vi "S4GUI.vi"() -> ()   [LabVIEW 2018] (continued)
            n2694 = call-dynamic "Read AcquisitionA.vi"("error in (no error)"=w6516, "S4ACS_GUI in"=w6518) -> ("error out"=w6521:errorcluster, "Acquisition.lvclass"=w6520:refnum<class "Acquisition.lvclass">, "S4ACS_GUI out"=w6517:refnum<class "S4GUI.lvclass">)  [unwired: 7 in]
            n2695 = call-dynamic "Read Channel.vi"("error in (no error)"=w6521, "Acquisition in"=w6520) -> ("error out"=w6523:errorcluster, "Channel.lvclass"=w6522:refnum<class "Channel.lvclass">, "Acquisition out"=w6529:refnum<class "Acquisition.lvclass">)  [unwired: 7 in]
            n2696 = call-dynamic "Read State Machine.vi"("error in (no error)"=w6523, "Device in"=w6522) -> ("error out"=w6525:errorcluster, "State Machine.lvclass"=w6524:refnum<class "State Machine.lvclass">, "Device out"=w6527:refnum<class "Channel.lvclass">)  [unwired: 7 in]
            n2697 = call "Next State.vi"("error in (no error)"=w6525, "New_State"=u32 80, "State Machine in"=w6524) -> ("error out"=w6528:errorcluster, "State Machine out"=w6526:refnum<class "State Machine.lvclass">)  [unwired: 7 in]
            n2698 = call-dynamic "Write State Machine.vi"("error in (no error)"=w6528, "State Machine.lvclass"=w6526, "Device in"=w6527) -> ("error out"=w6530:errorcluster, "Device out"=w6531:refnum<class "Channel.lvclass">)  [unwired: 7 in]
            n2699 = call-dynamic "Write Channel.vi"("error in (no error)"=w6530, "Channel.lvclass"=w6531, "Acquisition in"=w6529) -> ("error out"=w6513:errorcluster, "Acquisition out"=w6514:refnum<class "Acquisition.lvclass">)  [unwired: 7 in]
            n2700 = call-dynamic "Write Acq_state.vi"("error in (no error)"=w6513, "Acq_state"=u32 0, "Acquisition in"=w6514) -> ("error out"=w6512:errorcluster, "Acquisition out"=w6511:refnum<class "Acquisition.lvclass">)  [unwired: 7 in]
            n2701 = call-dynamic "Write AcquisitionA.vi"("error in (no error)"=w6512, "Acquisition.lvclass"=w6511, "S4ACS_GUI in"=w6517) -> ("error out"=w6499:errorcluster, "S4ACS_GUI out"=w6497:refnum<class "S4GUI.lvclass">)  [unwired: 7 in]
            n2702 = call "Read Instrument.lvclass.vi"("error in (no error)"=w6499, "S4ACS_GUI in"=w6497) -> ("error out"=w6506:errorcluster, "Instrument.lvclass"=w6509:refnum<class "Instrument.lvclass">, "S4ACS_GUI out"=w6510:refnum<class "S4GUI.lvclass">)  [unwired: 7 in]
            n2703 = call "Read WPROT.vi"("error in (no error)"=w6506, "Instrument in"=w6509) -> ("error out"=w6505:errorcluster, "Opt_Selector.lvclass"=w6507:refnum<class "Opt_Selector.lvclass">, "Instrument out"=w6508:refnum<class "Instrument.lvclass">)  [unwired: 7 in]
            n2704 = call-dynamic "Read sequencia_ant.vi"("error in (no error)"=w6505, "Opt_Selector in"=w6507) -> ("error out"=w6501:errorcluster, "sequencia_ant"=w6500:u16, "Opt_Selector out"=w6502:refnum<class "Opt_Selector.lvclass">)  [unwired: 7 in]
            n2705 = call-dynamic "Write sequencia.vi"("error in (no error)"=w6501, "sequencia"=w6500, "Opt_Selector in"=w6502) -> ("error out"=w6490:errorcluster, "Opt_Selector out"=w6491:refnum<class "Opt_Selector.lvclass">)  [unwired: 7 in]
            n2706 = call-dynamic "Read State Machine.vi"("error in (no error)"=w6490, "Device in"=w6491) -> ("error out"=w6493:errorcluster, "State Machine.lvclass"=w6496:refnum<class "State Machine.lvclass">, "Device out"=w6489:refnum<class "Opt_Selector.lvclass">)  [unwired: 7 in]
            n2707 = call "Next State.vi"("error in (no error)"=w6493, "New_State"=10, "State Machine in"=w6496) -> ("error out"=w6492:errorcluster, "State Machine out"=w6495:refnum<class "State Machine.lvclass">)  [unwired: 7 in]
            n2708 = call-dynamic "Write State Machine.vi"("error in (no error)"=w6492, "State Machine.lvclass"=w6495, "Device in"=w6489) -> ("error out"=w6487:errorcluster, "Device out"=w6488:refnum<class "Opt_Selector.lvclass">)  [unwired: 7 in]
            n2709 = call "Write WPROT.vi"("error in (no error)"=w6487, "Opt_Selector.lvclass"=w6488, "Instrument in"=w6508) -> ("error out"=w6504:errorcluster, "Instrument out"=w6503:refnum<class "Instrument.lvclass">)  [unwired: 7 in]
            n2710 = call "Write Instrument.lvclass.vi"("error in (no error)"=w6504, "Instrument.lvclass"=w6503, "S4ACS_GUI in"=w6510) -> ("error out"=w6498:errorcluster, "S4ACS_GUI out"=w6486:refnum<class "S4GUI.lvclass">)  [unwired: 7 in]
          }
          frame Enabled {
            w6535 = FALSE ("Wait Until Done")
            n2711 = call <vilib>:"Application Directory.vi"() -> ("Application Directory"=w6538:path)
            n2712 = Build Path(base path=w6538, name or relative path="MsgAbort1.vi") -> (appended path=w6539:path)
            n2713 = Open VI Reference(vi path=w6539, error in (no error)=w6533) -> (vi reference=w6537:refnum<vi>, error out=w6536:errorcluster)  [unwired: 4 in]
            n2714 = invoke class="VI" method="Run VI"(reference=w6537, error in=w6536, "Wait until done"=w6535, "Auto Dispose Ref"=w6535) -> (error out=w6532:errorcluster)  [unwired: 1 in, 4 out]
          }
        }
      }
      event "Abort ch2": Value Change {
        n2715 = event-data() -> ()  [unwired: 1 in, 6 out]
        n2716 = disable-structure shown="Enabled" {
          disable-tunnel: w6544 -> [w6577 w6592]
          disable-tunnel: w6543 -> [w6575 w6593]
          disable-tunnel: [w6557 w6591] -> w6542
          disable-tunnel: [w6545 w6592] -> w6541
          frame Disabled {
            # "Para movimento \nda lamina retardadora"
            # "Restaura a última sequência de lâminas"
            n2717 = call "Read AcquisitionB.vi"("error in (no error)"=w6575, "S4ACS_GUI in"=w6577) -> ("error out"=w6580:errorcluster, "Acquisition.lvclass"=w6579:refnum<class "Acquisition.lvclass">, "S4ACS_GUI out"=w6576:refnum<class "S4GUI.lvclass">)  [unwired: 7 in]
            n2718 = call-dynamic "Read Channel.vi"("error in (no error)"=w6580, "Acquisition in"=w6579) -> ("error out"=w6582:errorcluster, "Channel.lvclass"=w6581:refnum<class "Channel.lvclass">, "Acquisition out"=w6588:refnum<class "Acquisition.lvclass">)  [unwired: 7 in]
            n2719 = call-dynamic "Read State Machine.vi"("error in (no error)"=w6582, "Device in"=w6581) -> ("error out"=w6584:errorcluster, "State Machine.lvclass"=w6583:refnum<class "State Machine.lvclass">, "Device out"=w6586:refnum<class "Channel.lvclass">)  [unwired: 7 in]
            n2720 = call "Next State.vi"("error in (no error)"=w6584, "New_State"=u32 80, "State Machine in"=w6583) -> ("error out"=w6587:errorcluster, "State Machine out"=w6585:refnum<class "State Machine.lvclass">)  [unwired: 7 in]
            n2721 = call-dynamic "Write State Machine.vi"("error in (no error)"=w6587, "State Machine.lvclass"=w6585, "Device in"=w6586) -> ("error out"=w6589:errorcluster, "Device out"=w6590:refnum<class "Channel.lvclass">)  [unwired: 7 in]
            n2722 = call-dynamic "Write Channel.vi"("error in (no error)"=w6589, "Channel.lvclass"=w6590, "Acquisition in"=w6588) -> ("error out"=w6572:errorcluster, "Acquisition out"=w6573:refnum<class "Acquisition.lvclass">)  [unwired: 7 in]
            n2723 = call-dynamic "Write Acq_state.vi"("error in (no error)"=w6572, "Acq_state"=u32 0, "Acquisition in"=w6573) -> ("error out"=w6571:errorcluster, "Acquisition out"=w6570:refnum<class "Acquisition.lvclass">)  [unwired: 7 in]
            n2724 = call "Write AcquisitionB.vi"("error in (no error)"=w6571, "Acquisition.lvclass"=w6570, "S4ACS_GUI in"=w6576) -> ("error out"=w6558:errorcluster, "S4ACS_GUI out"=w6556:refnum<class "S4GUI.lvclass">)  [unwired: 7 in]
            n2725 = call "Read Instrument.lvclass.vi"("error in (no error)"=w6558, "S4ACS_GUI in"=w6556) -> ("error out"=w6565:errorcluster, "Instrument.lvclass"=w6568:refnum<class "Instrument.lvclass">, "S4ACS_GUI out"=w6569:refnum<class "S4GUI.lvclass">)  [unwired: 7 in]
            n2726 = call "Read WPROT.vi"("error in (no error)"=w6565, "Instrument in"=w6568) -> ("error out"=w6564:errorcluster, "Opt_Selector.lvclass"=w6566:refnum<class "Opt_Selector.lvclass">, "Instrument out"=w6567:refnum<class "Instrument.lvclass">)  [unwired: 7 in]
            n2727 = call-dynamic "Read sequencia_ant.vi"("error in (no error)"=w6564, "Opt_Selector in"=w6566) -> ("error out"=w6560:errorcluster, "sequencia_ant"=w6559:u16, "Opt_Selector out"=w6561:refnum<class "Opt_Selector.lvclass">)  [unwired: 7 in]
            n2728 = call-dynamic "Write sequencia.vi"("error in (no error)"=w6560, "sequencia"=w6559, "Opt_Selector in"=w6561) -> ("error out"=w6549:errorcluster, "Opt_Selector out"=w6550:refnum<class "Opt_Selector.lvclass">)  [unwired: 7 in]
            n2729 = call-dynamic "Read State Machine.vi"("error in (no error)"=w6549, "Device in"=w6550) -> ("error out"=w6552:errorcluster, "State Machine.lvclass"=w6555:refnum<class "State Machine.lvclass">, "Device out"=w6548:refnum<class "Opt_Selector.lvclass">)  [unwired: 7 in]
            n2730 = call "Next State.vi"("error in (no error)"=w6552, "New_State"=10, "State Machine in"=w6555) -> ("error out"=w6551:errorcluster, "State Machine out"=w6554:refnum<class "State Machine.lvclass">)  [unwired: 7 in]
            n2731 = call-dynamic "Write State Machine.vi"("error in (no error)"=w6551, "State Machine.lvclass"=w6554, "Device in"=w6548) -> ("error out"=w6546:errorcluster, "Device out"=w6547:refnum<class "Opt_Selector.lvclass">)  [unwired: 7 in]
            n2732 = call "Write WPROT.vi"("error in (no error)"=w6546, "Opt_Selector.lvclass"=w6547, "Instrument in"=w6567) -> ("error out"=w6563:errorcluster, "Instrument out"=w6562:refnum<class "Instrument.lvclass">)  [unwired: 7 in]
            n2733 = call "Write Instrument.lvclass.vi"("error in (no error)"=w6563, "Instrument.lvclass"=w6562, "S4ACS_GUI in"=w6569) -> ("error out"=w6557:errorcluster, "S4ACS_GUI out"=w6545:refnum<class "S4GUI.lvclass">)  [unwired: 7 in]
          }
          frame Enabled {
            w6595 = FALSE ("Wait Until Done")
            n2734 = call <vilib>:"Application Directory.vi"() -> ("Application Directory"=w6598:path)
            n2735 = Build Path(base path=w6598, name or relative path="MsgAbort2.vi") -> (appended path=w6599:path)
            n2736 = Open VI Reference(vi path=w6599, error in (no error)=w6593) -> (vi reference=w6597:refnum<vi>, error out=w6596:errorcluster)  [unwired: 4 in]
            n2737 = invoke class="VI" method="Run VI"(reference=w6597, error in=w6596, "Wait until done"=w6595, "Auto Dispose Ref"=w6595) -> (error out=w6591:errorcluster)  [unwired: 1 in, 4 out]
          }
        }
      }
      event "Abort ch3": Value Change {
        n2738 = event-data() -> ()  [unwired: 1 in, 6 out]
        n2739 = disable-structure shown="Enabled" {
          disable-tunnel: w6603 -> [w6636 w6651]
          disable-tunnel: w6602 -> [w6634 w6652]
          disable-tunnel: [w6616 w6650] -> w6601
          disable-tunnel: [w6604 w6651] -> w6600
          frame Disabled {
            # "Para movimento \nda lamina retardadora"
            # "Restaura a última sequência de lâminas"
            n2740 = call-dynamic "Read AcquisitionC.vi"("error in (no error)"=w6634, "S4ACS_GUI in"=w6636) -> ("error out"=w6639:errorcluster, "Acquisition.lvclass"=w6638:refnum<class "Acquisition.lvclass">, "S4ACS_GUI out"=w6635:refnum<class "S4GUI.lvclass">)  [unwired: 7 in]
            n2741 = call-dynamic "Read Channel.vi"("error in (no error)"=w6639, "Acquisition in"=w6638) -> ("error out"=w6641:errorcluster, "Channel.lvclass"=w6640:refnum<class "Channel.lvclass">, "Acquisition out"=w6647:refnum<class "Acquisition.lvclass">)  [unwired: 7 in]
            n2742 = call-dynamic "Read State Machine.vi"("error in (no error)"=w6641, "Device in"=w6640) -> ("error out"=w6643:errorcluster, "State Machine.lvclass"=w6642:refnum<class "State Machine.lvclass">, "Device out"=w6645:refnum<class "Channel.lvclass">)  [unwired: 7 in]
            n2743 = call "Next State.vi"("error in (no error)"=w6643, "New_State"=u32 80, "State Machine in"=w6642) -> ("error out"=w6646:errorcluster, "State Machine out"=w6644:refnum<class "State Machine.lvclass">)  [unwired: 7 in]
            n2744 = call-dynamic "Write State Machine.vi"("error in (no error)"=w6646, "State Machine.lvclass"=w6644, "Device in"=w6645) -> ("error out"=w6648:errorcluster, "Device out"=w6649:refnum<class "Channel.lvclass">)  [unwired: 7 in]
            n2745 = call-dynamic "Write Channel.vi"("error in (no error)"=w6648, "Channel.lvclass"=w6649, "Acquisition in"=w6647) -> ("error out"=w6631:errorcluster, "Acquisition out"=w6632:refnum<class "Acquisition.lvclass">)  [unwired: 7 in]
            n2746 = call-dynamic "Write Acq_state.vi"("error in (no error)"=w6631, "Acq_state"=u32 0, "Acquisition in"=w6632) -> ("error out"=w6630:errorcluster, "Acquisition out"=w6629:refnum<class "Acquisition.lvclass">)  [unwired: 7 in]
            n2747 = call-dynamic "Write AcquisitionC.vi"("error in (no error)"=w6630, "Acquisition.lvclass"=w6629, "S4ACS_GUI in"=w6635) -> ("error out"=w6617:errorcluster, "S4ACS_GUI out"=w6615:refnum<class "S4GUI.lvclass">)  [unwired: 7 in]
            n2748 = call "Read Instrument.lvclass.vi"("error in (no error)"=w6617, "S4ACS_GUI in"=w6615) -> ("error out"=w6624:errorcluster, "Instrument.lvclass"=w6627:refnum<class "Instrument.lvclass">, "S4ACS_GUI out"=w6628:refnum<class "S4GUI.lvclass">)  [unwired: 7 in]
            n2749 = call "Read WPROT.vi"("error in (no error)"=w6624, "Instrument in"=w6627) -> ("error out"=w6623:errorcluster, "Opt_Selector.lvclass"=w6625:refnum<class "Opt_Selector.lvclass">, "Instrument out"=w6626:refnum<class "Instrument.lvclass">)  [unwired: 7 in]
            n2750 = call-dynamic "Read sequencia_ant.vi"("error in (no error)"=w6623, "Opt_Selector in"=w6625) -> ("error out"=w6619:errorcluster, "sequencia_ant"=w6618:u16, "Opt_Selector out"=w6620:refnum<class "Opt_Selector.lvclass">)  [unwired: 7 in]
            n2751 = call-dynamic "Write sequencia.vi"("error in (no error)"=w6619, "sequencia"=w6618, "Opt_Selector in"=w6620) -> ("error out"=w6608:errorcluster, "Opt_Selector out"=w6609:refnum<class "Opt_Selector.lvclass">)  [unwired: 7 in]
            n2752 = call-dynamic "Read State Machine.vi"("error in (no error)"=w6608, "Device in"=w6609) -> ("error out"=w6611:errorcluster, "State Machine.lvclass"=w6614:refnum<class "State Machine.lvclass">, "Device out"=w6607:refnum<class "Opt_Selector.lvclass">)  [unwired: 7 in]
            n2753 = call "Next State.vi"("error in (no error)"=w6611, "New_State"=10, "State Machine in"=w6614) -> ("error out"=w6610:errorcluster, "State Machine out"=w6613:refnum<class "State Machine.lvclass">)  [unwired: 7 in]
            n2754 = call-dynamic "Write State Machine.vi"("error in (no error)"=w6610, "State Machine.lvclass"=w6613, "Device in"=w6607) -> ("error out"=w6605:errorcluster, "Device out"=w6606:refnum<class "Opt_Selector.lvclass">)  [unwired: 7 in]
            n2755 = call "Write WPROT.vi"("error in (no error)"=w6605, "Opt_Selector.lvclass"=w6606, "Instrument in"=w6626) -> ("error out"=w6622:errorcluster, "Instrument out"=w6621:refnum<class "Instrument.lvclass">)  [unwired: 7 in]
            n2756 = call "Write Instrument.lvclass.vi"("error in (no error)"=w6622, "Instrument.lvclass"=w6621, "S4ACS_GUI in"=w6628) -> ("error out"=w6616:errorcluster, "S4ACS_GUI out"=w6604:refnum<class "S4GUI.lvclass">)  [unwired: 7 in]
          }
          frame Enabled {
            w6654 = FALSE ("Wait Until Done")
            n2757 = call <vilib>:"Application Directory.vi"() -> ("Application Directory"=w6657:path)
            n2758 = Build Path(base path=w6657, name or relative path="MsgAbort3.vi") -> (appended path=w6658:path)
            n2759 = Open VI Reference(vi path=w6658, error in (no error)=w6652) -> (vi reference=w6656:refnum<vi>, error out=w6655:errorcluster)  [unwired: 4 in]
            n2760 = invoke class="VI" method="Run VI"(reference=w6656, error in=w6655, "Wait until done"=w6654, "Auto Dispose Ref"=w6654) -> (error out=w6650:errorcluster)  [unwired: 1 in, 4 out]
          }
        }
      }
      event "Abort ch4": Value Change {
        n2761 = event-data() -> ()  [unwired: 1 in, 6 out]
        n2762 = disable-structure shown="Enabled" {
          disable-tunnel: w6662 -> [w6695 w6710]
          disable-tunnel: w6661 -> [w6693 w6711]
          disable-tunnel: [w6675 w6709] -> w6660
          disable-tunnel: [w6663 w6710] -> w6659
          frame Disabled {
            # "Para movimento \nda lamina retardadora"
            # "Restaura a última sequência de lâminas"
            n2763 = call-dynamic "Read AcquisitionD.vi"("error in (no error)"=w6693, "S4ACS_GUI in"=w6695) -> ("error out"=w6698:errorcluster, "Acquisition.lvclass"=w6697:refnum<class "Acquisition.lvclass">, "S4ACS_GUI out"=w6694:refnum<class "S4GUI.lvclass">)  [unwired: 7 in]
            n2764 = call-dynamic "Read Channel.vi"("error in (no error)"=w6698, "Acquisition in"=w6697) -> ("error out"=w6700:errorcluster, "Channel.lvclass"=w6699:refnum<class "Channel.lvclass">, "Acquisition out"=w6706:refnum<class "Acquisition.lvclass">)  [unwired: 7 in]
            n2765 = call-dynamic "Read State Machine.vi"("error in (no error)"=w6700, "Device in"=w6699) -> ("error out"=w6702:errorcluster, "State Machine.lvclass"=w6701:refnum<class "State Machine.lvclass">, "Device out"=w6704:refnum<class "Channel.lvclass">)  [unwired: 7 in]
            n2766 = call "Next State.vi"("error in (no error)"=w6702, "New_State"=u32 80, "State Machine in"=w6701) -> ("error out"=w6705:errorcluster, "State Machine out"=w6703:refnum<class "State Machine.lvclass">)  [unwired: 7 in]
            n2767 = call-dynamic "Write State Machine.vi"("error in (no error)"=w6705, "State Machine.lvclass"=w6703, "Device in"=w6704) -> ("error out"=w6707:errorcluster, "Device out"=w6708:refnum<class "Channel.lvclass">)  [unwired: 7 in]
            n2768 = call-dynamic "Write Channel.vi"("error in (no error)"=w6707, "Channel.lvclass"=w6708, "Acquisition in"=w6706) -> ("error out"=w6690:errorcluster, "Acquisition out"=w6691:refnum<class "Acquisition.lvclass">)  [unwired: 7 in]
            n2769 = call-dynamic "Write Acq_state.vi"("error in (no error)"=w6690, "Acq_state"=u32 0, "Acquisition in"=w6691) -> ("error out"=w6689:errorcluster, "Acquisition out"=w6688:refnum<class "Acquisition.lvclass">)  [unwired: 7 in]
            n2770 = call-dynamic "Write AcquisitionD.vi"("error in (no error)"=w6689, "Acquisition.lvclass"=w6688, "S4ACS_GUI in"=w6694) -> ("error out"=w6676:errorcluster, "S4ACS_GUI out"=w6674:refnum<class "S4GUI.lvclass">)  [unwired: 7 in]
            n2771 = call "Read Instrument.lvclass.vi"("error in (no error)"=w6676, "S4ACS_GUI in"=w6674) -> ("error out"=w6683:errorcluster, "Instrument.lvclass"=w6686:refnum<class "Instrument.lvclass">, "S4ACS_GUI out"=w6687:refnum<class "S4GUI.lvclass">)  [unwired: 7 in]
            n2772 = call "Read WPROT.vi"("error in (no error)"=w6683, "Instrument in"=w6686) -> ("error out"=w6682:errorcluster, "Opt_Selector.lvclass"=w6684:refnum<class "Opt_Selector.lvclass">, "Instrument out"=w6685:refnum<class "Instrument.lvclass">)  [unwired: 7 in]
            n2773 = call-dynamic "Read sequencia_ant.vi"("error in (no error)"=w6682, "Opt_Selector in"=w6684) -> ("error out"=w6678:errorcluster, "sequencia_ant"=w6677:u16, "Opt_Selector out"=w6679:refnum<class "Opt_Selector.lvclass">)  [unwired: 7 in]
            n2774 = call-dynamic "Write sequencia.vi"("error in (no error)"=w6678, "sequencia"=w6677, "Opt_Selector in"=w6679) -> ("error out"=w6667:errorcluster, "Opt_Selector out"=w6668:refnum<class "Opt_Selector.lvclass">)  [unwired: 7 in]
            n2775 = call-dynamic "Read State Machine.vi"("error in (no error)"=w6667, "Device in"=w6668) -> ("error out"=w6670:errorcluster, "State Machine.lvclass"=w6673:refnum<class "State Machine.lvclass">, "Device out"=w6666:refnum<class "Opt_Selector.lvclass">)  [unwired: 7 in]
            n2776 = call "Next State.vi"("error in (no error)"=w6670, "New_State"=10, "State Machine in"=w6673) -> ("error out"=w6669:errorcluster, "State Machine out"=w6672:refnum<class "State Machine.lvclass">)  [unwired: 7 in]
            n2777 = call-dynamic "Write State Machine.vi"("error in (no error)"=w6669, "State Machine.lvclass"=w6672, "Device in"=w6666) -> ("error out"=w6664:errorcluster, "Device out"=w6665:refnum<class "Opt_Selector.lvclass">)  [unwired: 7 in]
            n2778 = call "Write WPROT.vi"("error in (no error)"=w6664, "Opt_Selector.lvclass"=w6665, "Instrument in"=w6685) -> ("error out"=w6681:errorcluster, "Instrument out"=w6680:refnum<class "Instrument.lvclass">)  [unwired: 7 in]
            n2779 = call "Write Instrument.lvclass.vi"("error in (no error)"=w6681, "Instrument.lvclass"=w6680, "S4ACS_GUI in"=w6687) -> ("error out"=w6675:errorcluster, "S4ACS_GUI out"=w6663:refnum<class "S4GUI.lvclass">)  [unwired: 7 in]
          }
          frame Enabled {
            w6713 = FALSE ("Wait Until Done")
            n2780 = call <vilib>:"Application Directory.vi"() -> ("Application Directory"=w6716:path)
            n2781 = Build Path(base path=w6716, name or relative path="MsgAbort4.vi") -> (appended path=w6717:path)
            n2782 = Open VI Reference(vi path=w6717, error in (no error)=w6711) -> (vi reference=w6715:refnum<vi>, error out=w6714:errorcluster)  [unwired: 4 in]
            n2783 = invoke class="VI" method="Run VI"(reference=w6715, error in=w6714, "Wait until done"=w6713, "Auto Dispose Ref"=w6713) -> (error out=w6709:errorcluster)  [unwired: 1 in, 4 out]
          }
        }
      }
      event "Exposure Time": Value Change {
        n2784 = event-data() -> ()  [unwired: 1 in, 4 out]
        n2785 = call-dynamic "Read AcquisitionA.vi"("error in (no error)"=w6736, "S4ACS_GUI in"=w6737) -> ("error out"=w6734:errorcluster, "Acquisition.lvclass"=w6735:refnum<class "Acquisition.lvclass">, "S4ACS_GUI out"=w6731:refnum<class "S4GUI.lvclass">)  [unwired: 7 in]
        n2786 = call-dynamic "Read Channel.vi"("error in (no error)"=w6734, "Acquisition in"=w6735) -> ("error out"=w6720:errorcluster, "Channel.lvclass"=w6721:refnum<class "Channel.lvclass">, "Acquisition out"=w6733:refnum<class "Acquisition.lvclass">)  [unwired: 7 in]
        n2787 = call-dynamic "Read Interface.vi"("error in (no error)"=w6720, "Channel in"=w6721) -> ("error out"=w6727:errorcluster, "Interface.lvclass"=w6728:refnum<class "Interface.lvclass">, "Channel out"=w6725:refnum<class "Channel.lvclass">)  [unwired: 7 in]
        n2788 = call "Write Exposure Time.vi"("error in (no error)"=w6727, "Exposure Time"="Exposure Time", "Interface in"=w6728) -> ("error out"=w6722:errorcluster, "Interface out"=w6726:refnum<class "Interface.lvclass">)  [unwired: 7 in]
        n2789 = call-dynamic "Write Interface.vi"("error in (no error)"=w6722, "Interface.lvclass"=w6726, "Channel in"=w6725) -> ("error out"=w6723:errorcluster, "Channel out"=w6724:refnum<class "Channel.lvclass">)  [unwired: 7 in]
        n2790 = call-dynamic "Write Channel.vi"("error in (no error)"=w6723, "Channel.lvclass"=w6724, "Acquisition in"=w6733) -> ("error out"=w6730:errorcluster, "Acquisition out"=w6732:refnum<class "Acquisition.lvclass">)  [unwired: 7 in]
        n2791 = call-dynamic "Write AcquisitionA.vi"("error in (no error)"=w6730, "Acquisition.lvclass"=w6732, "S4ACS_GUI in"=w6731) -> ("error out"=w6729:errorcluster, "S4ACS_GUI out"=w6718:refnum<class "S4GUI.lvclass">)  [unwired: 7 in]
      }
      event "SyncBox": Value Change {
        n2792 = event-data() -> ()  [unwired: 1 in, 4 out]
        n2793 = call-dynamic "Read Sync Box.lvclass.vi"("error in (no error)"=w6740, "SPARC4_AC in"=w6741) -> ("error out"=w6756:errorcluster, "Sync Box.lvclass"=w6757:refnum<class "Sync Box.lvclass">, "SPARC4_AC out"=w6745:refnum<class "S4GUI.lvclass">)  [unwired: 7 in]
        n2794 = call-dynamic "Read Trigger.lvclass.vi"("error in (no error)"=w6756, "Sync Box in"=w6757) -> ("error out"=w6754:errorcluster, "Trigger.lvclass"=w6755:refnum<class "Trigger.lvclass">, "Sync Box out"=w6748:refnum<class "Sync Box.lvclass">)  [unwired: 7 in]
        n2795 = call-dynamic "Read State Machine.vi"("error in (no error)"=w6754, "Device in"=w6755) -> ("error out"=w6752:errorcluster, "State Machine.lvclass"=w6753:refnum<class "State Machine.lvclass">, "Device out"=w6749:refnum<class "Trigger.lvclass">)  [unwired: 7 in]
        n2796 = call "Next State.vi"("error in (no error)"=w6752, "New_State"=u32 1, "State Machine in"=w6753) -> ("error out"=w6747:errorcluster, "State Machine out"=w6750:refnum<class "State Machine.lvclass">)  [unwired: 7 in]
        n2797 = call-dynamic "Write State Machine.vi"("error in (no error)"=w6747, "State Machine.lvclass"=w6750, "Device in"=w6749) -> ("error out"=w6743:errorcluster, "Device out"=w6742:refnum<class "Trigger.lvclass">)  [unwired: 7 in]
        n2798 = call-dynamic "Write Trigger.lvclass.vi"("error in (no error)"=w6743, "Trigger.lvclass"=w6742, "Sync Box in"=w6748) -> ("error out"=w6744:errorcluster, "Sync Box out"=w6746:refnum<class "Sync Box.lvclass">)  [unwired: 7 in]
        n2799 = call-dynamic "Write Sync Box.lvclass.vi"("error in (no error)"=w6744, "Sync Box.lvclass"=w6746, "SPARC4_AC in"=w6745) -> ("error out"=w6739:errorcluster, "SPARC4_AC out"=w6738:refnum<class "S4GUI.lvclass">)  [unwired: 7 in]
      }
      event "Fire manual", "Fire": Value Change {
        n2800 = event-data() -> ()  [unwired: 1 in, 4 out]
        n2801 = call-dynamic "Read Sync Box.lvclass.vi"("error in (no error)"=w6760, "SPARC4_AC in"=w6761) -> ("error out"=w6776:errorcluster, "Sync Box.lvclass"=w6777:refnum<class "Sync Box.lvclass">, "SPARC4_AC out"=w6765:refnum<class "S4GUI.lvclass">)  [unwired: 7 in]
        n2802 = call-dynamic "Read Trigger.lvclass.vi"("error in (no error)"=w6776, "Sync Box in"=w6777) -> ("error out"=w6774:errorcluster, "Trigger.lvclass"=w6775:refnum<class "Trigger.lvclass">, "Sync Box out"=w6768:refnum<class "Sync Box.lvclass">)  [unwired: 7 in]
        n2803 = call-dynamic "Read State Machine.vi"("error in (no error)"=w6774, "Device in"=w6775) -> ("error out"=w6772:errorcluster, "State Machine.lvclass"=w6773:refnum<class "State Machine.lvclass">, "Device out"=w6769:refnum<class "Trigger.lvclass">)  [unwired: 7 in]
        n2804 = call "Next State.vi"("error in (no error)"=w6772, "New_State"=u32 40, "State Machine in"=w6773) -> ("error out"=w6767:errorcluster, "State Machine out"=w6770:refnum<class "State Machine.lvclass">)  [unwired: 7 in]
        n2805 = call-dynamic "Write State Machine.vi"("error in (no error)"=w6767, "State Machine.lvclass"=w6770, "Device in"=w6769) -> ("error out"=w6763:errorcluster, "Device out"=w6762:refnum<class "Trigger.lvclass">)  [unwired: 7 in]
        n2806 = call-dynamic "Write Trigger.lvclass.vi"("error in (no error)"=w6763, "Trigger.lvclass"=w6762, "Sync Box in"=w6768) -> ("error out"=w6764:errorcluster, "Sync Box out"=w6766:refnum<class "Sync Box.lvclass">)  [unwired: 7 in]
        n2807 = call-dynamic "Write Sync Box.lvclass.vi"("error in (no error)"=w6764, "Sync Box.lvclass"=w6766, "SPARC4_AC in"=w6765) -> ("error out"=w6759:errorcluster, "SPARC4_AC out"=w6758:refnum<class "S4GUI.lvclass">)  [unwired: 7 in]
      }
      event "Select Trigger Mode": Value Change {
        n2808 = event-data() -> ("NewVal"=w6779:bool)  [unwired: 1 in, 2 out]
        n2809 = call-dynamic "Read Sync Box.lvclass.vi"("error in (no error)"=w6787, "SPARC4_AC in"=w6788) -> ("error out"=w6799:errorcluster, "Sync Box.lvclass"=w6800:refnum<class "Sync Box.lvclass">, "SPARC4_AC out"=w6792:refnum<class "S4GUI.lvclass">)  [unwired: 7 in]
        n2810 = call-dynamic "Read Trigger.lvclass.vi"("error in (no error)"=w6799, "Sync Box in"=w6800) -> ("error out"=w6780:errorcluster, "Trigger.lvclass"=w6783:refnum<class "Trigger.lvclass">, "Sync Box out"=w6795:refnum<class "Sync Box.lvclass">)  [unwired: 7 in]
        n2811 = call-dynamic "Write Trigger Mode Target.vi"("error in (no error)"=w6780, "Trigger Mode Target"=w6779, "Trigger in"=w6783) -> ("error out"=w6781:errorcluster, "Trigger out"=w6782:refnum<class "Trigger.lvclass">)  [unwired: 7 in]
        n2812 = call-dynamic "Read State Machine.vi"("error in (no error)"=w6781, "Device in"=w6782) -> ("error out"=w6784:errorcluster, "State Machine.lvclass"=w6785:refnum<class "State Machine.lvclass">, "Device out"=w6796:refnum<class "Trigger.lvclass">)  [unwired: 7 in]
        n2813 = call "Next State.vi"("error in (no error)"=w6784, "New_State"=u32 30, "State Machine in"=w6785) -> ("error out"=w6794:errorcluster, "State Machine out"=w6797:refnum<class "State Machine.lvclass">)  [unwired: 7 in]
        n2814 = call-dynamic "Write State Machine.vi"("error in (no error)"=w6794, "State Machine.lvclass"=w6797, "Device in"=w6796) -> ("error out"=w6790:errorcluster, "Device out"=w6789:refnum<class "Trigger.lvclass">)  [unwired: 7 in]
        n2815 = call-dynamic "Write Trigger.lvclass.vi"("error in (no error)"=w6790, "Trigger.lvclass"=w6789, "Sync Box in"=w6795) -> ("error out"=w6791:errorcluster, "Sync Box out"=w6793:refnum<class "Sync Box.lvclass">)  [unwired: 7 in]
        n2816 = call-dynamic "Write Sync Box.lvclass.vi"("error in (no error)"=w6791, "Sync Box.lvclass"=w6793, "SPARC4_AC in"=w6792) -> ("error out"=w6786:errorcluster, "SPARC4_AC out"=w6778:refnum<class "S4GUI.lvclass">)  [unwired: 7 in]
      }
      event "Set SyncBox": Value Change {
        n2817 = event-data() -> ()  [unwired: 1 in, 4 out]
        n2818 = call-dynamic "Read Sync Box.lvclass.vi"("error in (no error)"=w6803, "SPARC4_AC in"=w6804) -> ("error out"=w6819:errorcluster, "Sync Box.lvclass"=w6820:refnum<class "Sync Box.lvclass">, "SPARC4_AC out"=w6808:refnum<class "S4GUI.lvclass">)  [unwired: 7 in]
        n2819 = call-dynamic "Read Trigger.lvclass.vi"("error in (no error)"=w6819, "Sync Box in"=w6820) -> ("error out"=w6817:errorcluster, "Trigger.lvclass"=w6818:refnum<class "Trigger.lvclass">, "Sync Box out"=w6811:refnum<class "Sync Box.lvclass">)  [unwired: 7 in]
        n2820 = call-dynamic "Read State Machine.vi"("error in (no error)"=w6817, "Device in"=w6818) -> ("error out"=w6815:errorcluster, "State Machine.lvclass"=w6816:refnum<class "State Machine.lvclass">, "Device out"=w6812:refnum<class "Trigger.lvclass">)  [unwired: 7 in]
        n2821 = call "Next State.vi"("error in (no error)"=w6815, "New_State"=u32 10, "State Machine in"=w6816) -> ("error out"=w6810:errorcluster, "State Machine out"=w6813:refnum<class "State Machine.lvclass">)  [unwired: 7 in]
        n2822 = call-dynamic "Write State Machine.vi"("error in (no error)"=w6810, "State Machine.lvclass"=w6813, "Device in"=w6812) -> ("error out"=w6806:errorcluster, "Device out"=w6805:refnum<class "Trigger.lvclass">)  [unwired: 7 in]
        n2823 = call-dynamic "Write Trigger.lvclass.vi"("error in (no error)"=w6806, "Trigger.lvclass"=w6805, "Sync Box in"=w6811) -> ("error out"=w6807:errorcluster, "Sync Box out"=w6809:refnum<class "Sync Box.lvclass">)  [unwired: 7 in]
        n2824 = call-dynamic "Write Sync Box.lvclass.vi"("error in (no error)"=w6807, "Sync Box.lvclass"=w6809, "SPARC4_AC in"=w6808) -> ("error out"=w6802:errorcluster, "SPARC4_AC out"=w6801:refnum<class "S4GUI.lvclass">)  [unwired: 7 in]
      }
      event "Cooler 1": Value Change {
        n2825 = event-data() -> ("NewVal"=w6821:bool)  [unwired: 1 in]
        n2826 = case shown="True" w6821 {
          tunnel: w6825 -> [w6827 w6831]
          tunnel: w6824 -> [w6826 w6830]
          tunnel: [w6826 w6829] -> w6823
          tunnel: [w6827 w6828] -> w6822
          frame False {
          }
          frame True {
            n2827 = call-dynamic "Read AcquisitionA.vi"("error in (no error)"=w6830, "S4ACS_GUI in"=w6831) -> ("error out"=w6846:errorcluster, "Acquisition.lvclass"=w6847:refnum<class "Acquisition.lvclass">, "S4ACS_GUI out"=w6835:refnum<class "S4GUI.lvclass">)  [unwired: 7 in]
            n2828 = call-dynamic "Read Channel.vi"("error in (no error)"=w6846, "Acquisition in"=w6847) -> ("error out"=w6844:errorcluster, "Channel.lvclass"=w6845:refnum<class "Channel.lvclass">, "Acquisition out"=w6838:refnum<class "Acquisition.lvclass">)  [unwired: 7 in]
            n2829 = call-dynamic "Read State Machine.vi"("error in (no error)"=w6844, "Device in"=w6845) -> ("error out"=w6842:errorcluster, "State Machine.lvclass"=w6843:refnum<class "State Machine.lvclass">, "Device out"=w6839:refnum<class "Channel.lvclass">)  [unwired: 7 in]
            n2830 = call "Next State.vi"("error in (no error)"=w6842, "New_State"=u32 30, "State Machine in"=w6843) -> ("error out"=w6837:errorcluster, "State Machine out"=w6840:refnum<class "State Machine.lvclass">)  [unwired: 7 in]
            n2831 = call-dynamic "Write State Machine.vi"("error in (no error)"=w6837, "State Machine.lvclass"=w6840, "Device in"=w6839) -> ("error out"=w6833:errorcluster, "Device out"=w6832:refnum<class "Channel.lvclass">)  [unwired: 7 in]
            n2832 = call-dynamic "Write Channel.vi"("error in (no error)"=w6833, "Channel.lvclass"=w6832, "Acquisition in"=w6838) -> ("error out"=w6834:errorcluster, "Acquisition out"=w6836:refnum<class "Acquisition.lvclass">)  [unwired: 7 in]
            n2833 = call-dynamic "Write AcquisitionA.vi"("error in (no error)"=w6834, "Acquisition.lvclass"=w6836, "S4ACS_GUI in"=w6835) -> ("error out"=w6829:errorcluster, "S4ACS_GUI out"=w6828:refnum<class "S4GUI.lvclass">)  [unwired: 7 in]
          }
        }
      }
      event "Cooler 2": Value Change {
        n2834 = event-data() -> ("NewVal"=w6848:bool)  [unwired: 1 in]
        n2835 = case shown="True" w6848 {
          tunnel: w6852 -> [w6854 w6858]
          tunnel: w6851 -> [w6853 w6857]
          tunnel: [w6853 w6856] -> w6850
          tunnel: [w6854 w6855] -> w6849
          frame False {
          }
          frame True {
            n2836 = call "Read AcquisitionB.vi"("error in (no error)"=w6857, "S4ACS_GUI in"=w6858) -> ("error out"=w6873:errorcluster, "Acquisition.lvclass"=w6874:refnum<class "Acquisition.lvclass">, "S4ACS_GUI out"=w6862:refnum<class "S4GUI.lvclass">)  [unwired: 7 in]
            n2837 = call-dynamic "Read Channel.vi"("error in (no error)"=w6873, "Acquisition in"=w6874) -> ("error out"=w6871:errorcluster, "Channel.lvclass"=w6872:refnum<class "Channel.lvclass">, "Acquisition out"=w6865:refnum<class "Acquisition.lvclass">)  [unwired: 7 in]
            n2838 = call-dynamic "Read State Machine.vi"("error in (no error)"=w6871, "Device in"=w6872) -> ("error out"=w6869:errorcluster, "State Machine.lvclass"=w6870:refnum<class "State Machine.lvclass">, "Device out"=w6866:refnum<class "Channel.lvclass">)  [unwired: 7 in]
            n2839 = call "Next State.vi"("error in (no error)"=w6869, "New_State"=u32 30, "State Machine in"=w6870) -> ("error out"=w6864:errorcluster, "State Machine out"=w6867:refnum<class "State Machine.lvclass">)  [unwired: 7 in]
            n2840 = call-dynamic "Write State Machine.vi"("error in (no error)"=w6864, "State Machine.lvclass"=w6867, "Device in"=w6866) -> ("error out"=w6860:errorcluster, "Device out"=w6859:refnum<class "Channel.lvclass">)  [unwired: 7 in]
            n2841 = call-dynamic "Write Channel.vi"("error in (no error)"=w6860, "Channel.lvclass"=w6859, "Acquisition in"=w6865) -> ("error out"=w6861:errorcluster, "Acquisition out"=w6863:refnum<class "Acquisition.lvclass">)  [unwired: 7 in]
            n2842 = call "Write AcquisitionB.vi"("error in (no error)"=w6861, "Acquisition.lvclass"=w6863, "S4ACS_GUI in"=w6862) -> ("error out"=w6856:errorcluster, "S4ACS_GUI out"=w6855:refnum<class "S4GUI.lvclass">)  [unwired: 7 in]
          }
        }
      }
      event "Cooler 3": Value Change {
        n2843 = event-data() -> ("NewVal"=w6875:bool)  [unwired: 1 in]
        n2844 = case shown="True" w6875 {
          tunnel: w6879 -> [w6881 w6885]
          tunnel: w6878 -> [w6880 w6884]
          tunnel: [w6880 w6883] -> w6877
          tunnel: [w6881 w6882] -> w6876
          frame False {
          }
          frame True {
            n2845 = call-dynamic "Read AcquisitionC.vi"("error in (no error)"=w6884, "S4ACS_GUI in"=w6885) -> ("error out"=w6900:errorcluster, "Acquisition.lvclass"=w6901:refnum<class "Acquisition.lvclass">, "S4ACS_GUI out"=w6889:refnum<class "S4GUI.lvclass">)  [unwired: 7 in]
            n2846 = call-dynamic "Read Channel.vi"("error in (no error)"=w6900, "Acquisition in"=w6901) -> ("error out"=w6898:errorcluster, "Channel.lvclass"=w6899:refnum<class "Channel.lvclass">, "Acquisition out"=w6892:refnum<class "Acquisition.lvclass">)  [unwired: 7 in]
            n2847 = call-dynamic "Read State Machine.vi"("error in (no error)"=w6898, "Device in"=w6899) -> ("error out"=w6896:errorcluster, "State Machine.lvclass"=w6897:refnum<class "State Machine.lvclass">, "Device out"=w6893:refnum<class "Channel.lvclass">)  [unwired: 7 in]
            n2848 = call "Next State.vi"("error in (no error)"=w6896, "New_State"=u32 30, "State Machine in"=w6897) -> ("error out"=w6891:errorcluster, "State Machine out"=w6894:refnum<class "State Machine.lvclass">)  [unwired: 7 in]
            n2849 = call-dynamic "Write State Machine.vi"("error in (no error)"=w6891, "State Machine.lvclass"=w6894, "Device in"=w6893) -> ("error out"=w6887:errorcluster, "Device out"=w6886:refnum<class "Channel.lvclass">)  [unwired: 7 in]
            n2850 = call-dynamic "Write Channel.vi"("error in (no error)"=w6887, "Channel.lvclass"=w6886, "Acquisition in"=w6892) -> ("error out"=w6888:errorcluster, "Acquisition out"=w6890:refnum<class "Acquisition.lvclass">)  [unwired: 7 in]
            n2851 = call-dynamic "Write AcquisitionC.vi"("error in (no error)"=w6888, "Acquisition.lvclass"=w6890, "S4ACS_GUI in"=w6889) -> ("error out"=w6883:errorcluster, "S4ACS_GUI out"=w6882:refnum<class "S4GUI.lvclass">)  [unwired: 7 in]
          }
        }
      }
      event "Cooler 4": Value Change {
        n2852 = event-data() -> ("NewVal"=w6902:bool)  [unwired: 1 in]
        n2853 = case shown="True" w6902 {
          tunnel: w6906 -> [w6908 w6912]
          tunnel: w6905 -> [w6907 w6911]
          tunnel: [w6907 w6910] -> w6904
          tunnel: [w6908 w6909] -> w6903
          frame False {
          }
          frame True {
            n2854 = call-dynamic "Read AcquisitionD.vi"("error in (no error)"=w6911, "S4ACS_GUI in"=w6912) -> ("error out"=w6927:errorcluster, "Acquisition.lvclass"=w6928:refnum<class "Acquisition.lvclass">, "S4ACS_GUI out"=w6916:refnum<class "S4GUI.lvclass">)  [unwired: 7 in]
            n2855 = call-dynamic "Read Channel.vi"("error in (no error)"=w6927, "Acquisition in"=w6928) -> ("error out"=w6925:errorcluster, "Channel.lvclass"=w6926:refnum<class "Channel.lvclass">, "Acquisition out"=w6919:refnum<class "Acquisition.lvclass">)  [unwired: 7 in]
            n2856 = call-dynamic "Read State Machine.vi"("error in (no error)"=w6925, "Device in"=w6926) -> ("error out"=w6923:errorcluster, "State Machine.lvclass"=w6924:refnum<class "State Machine.lvclass">, "Device out"=w6920:refnum<class "Channel.lvclass">)  [unwired: 7 in]
            n2857 = call "Next State.vi"("error in (no error)"=w6923, "New_State"=u32 30, "State Machine in"=w6924) -> ("error out"=w6918:errorcluster, "State Machine out"=w6921:refnum<class "State Machine.lvclass">)  [unwired: 7 in]
            n2858 = call-dynamic "Write State Machine.vi"("error in (no error)"=w6918, "State Machine.lvclass"=w6921, "Device in"=w6920) -> ("error out"=w6914:errorcluster, "Device out"=w6913:refnum<class "Channel.lvclass">)  [unwired: 7 in]
            n2859 = call-dynamic "Write Channel.vi"("error in (no error)"=w6914, "Channel.lvclass"=w6913, "Acquisition in"=w6919) -> ("error out"=w6915:errorcluster, "Acquisition out"=w6917:refnum<class "Acquisition.lvclass">)  [unwired: 7 in]
            n2860 = call-dynamic "Write AcquisitionD.vi"("error in (no error)"=w6915, "Acquisition.lvclass"=w6917, "S4ACS_GUI in"=w6916) -> ("error out"=w6910:errorcluster, "S4ACS_GUI out"=w6909:refnum<class "S4GUI.lvclass">)  [unwired: 7 in]
          }
        }
      }
      event "Cooler status 4": Value Change {
        n2861 = event-data() -> ("NewVal"=w6929:bool)  [unwired: 1 in]
        n2862 = case shown="False" w6929 {
          tunnel: w6933 -> [w6942 w6955]
          tunnel: w6932 -> [w6941 w6954]
          tunnel: [w6940 w6954] -> w6931
          tunnel: [w6939 w6955] -> w6930
          frame False {
            n2863 = call-dynamic "Read AcquisitionD.vi"("error in (no error)"=w6941, "S4ACS_GUI in"=w6942) -> ("error out"=w6952:errorcluster, "Acquisition.lvclass"=w6953:refnum<class "Acquisition.lvclass">, "S4ACS_GUI out"=w6946:refnum<class "S4GUI.lvclass">)  [unwired: 7 in]
            n2864 = call-dynamic "Read Channel.vi"("error in (no error)"=w6952, "Acquisition in"=w6953) -> ("error out"=w6950:errorcluster, "Channel.lvclass"=w6951:refnum<class "Channel.lvclass">, "Acquisition out"=w6948:refnum<class "Acquisition.lvclass">)  [unwired: 7 in]
            n2865 = call-dynamic "Read State Machine.vi"("error in (no error)"=w6950, "Device in"=w6951) -> ("error out"=w6936:errorcluster, "State Machine.lvclass"=w6938:refnum<class "State Machine.lvclass">, "Device out"=w6949:refnum<class "Channel.lvclass">)  [unwired: 7 in]
            n2866 = call-dynamic "Read Previous State.vi"("error in (no error)"=w6936, "State Machine in"=w6938) -> ("error out"=w6935:errorcluster, "Previous State"=→"State":dbl, "State Machine out"=w6937:refnum<class "State Machine.lvclass">)  [unwired: 7 in]
            n2867 = call-dynamic "Write State Machine.vi"("error in (no error)"=w6935, "State Machine.lvclass"=w6937, "Device in"=w6949) -> ("error out"=w6944:errorcluster, "Device out"=w6943:refnum<class "Channel.lvclass">)  [unwired: 7 in]
            n2868 = call-dynamic "Write Channel.vi"("error in (no error)"=w6944, "Channel.lvclass"=w6943, "Acquisition in"=w6948) -> ("error out"=w6945:errorcluster, "Acquisition out"=w6947:refnum<class "Acquisition.lvclass">)  [unwired: 7 in]
            n2869 = call-dynamic "Write AcquisitionD.vi"("error in (no error)"=w6945, "Acquisition.lvclass"=w6947, "S4ACS_GUI in"=w6946) -> ("error out"=w6940:errorcluster, "S4ACS_GUI out"=w6939:refnum<class "S4GUI.lvclass">)  [unwired: 7 in]
          }
          frame True {
          }
        }
      }
      event "Set Temp 1": Value Change {
        n2870 = event-data() -> ("NewVal"=w6956:bool)  [unwired: 1 in]
        n2871 = case shown="True" w6956 {
          tunnel: w6960 -> [w6962 w6976]
          tunnel: w6959 -> [w6961 w6975]
          tunnel: [w6961 w6974] -> w6958
          tunnel: [w6962 w6973] -> w6957
          frame False {
          }
          frame True {
            n2872 = call-dynamic "Read AcquisitionA.vi"("error in (no error)"=w6975, "S4ACS_GUI in"=w6976) -> ("error out"=w6989:errorcluster, "Acquisition.lvclass"=w6990:refnum<class "Acquisition.lvclass">, "S4ACS_GUI out"=w6980:refnum<class "S4GUI.lvclass">)  [unwired: 7 in]
            n2873 = call-dynamic "Read Channel.vi"("error in (no error)"=w6989, "Acquisition in"=w6990) -> ("error out"=w6971:errorcluster, "Channel.lvclass"=w6972:refnum<class "Channel.lvclass">, "Acquisition out"=w6983:refnum<class "Acquisition.lvclass">)  [unwired: 7 in]
            n2874 = call-dynamic "Read Interface.vi"("error in (no error)"=w6971, "Channel in"=w6972) -> ("error out"=w6969:errorcluster, "Interface.lvclass"=w6970:refnum<class "Interface.lvclass">, "Channel out"=w6967:refnum<class "Channel.lvclass">)  [unwired: 7 in]
            n2875 = call-dynamic "Write Temperature.vi"("error in (no error)"=w6969, "Temperature"="Target Temp 1", "Interface in"=w6970) -> ("error out"=w6965:errorcluster, "Interface out"=w6968:refnum<class "Interface.lvclass">)  [unwired: 7 in]
            n2876 = call-dynamic "Write Interface.vi"("error in (no error)"=w6965, "Interface.lvclass"=w6968, "Channel in"=w6967) -> ("error out"=w6964:errorcluster, "Channel out"=w6966:refnum<class "Channel.lvclass">)  [unwired: 7 in]
            n2877 = call-dynamic "Read State Machine.vi"("error in (no error)"=w6964, "Device in"=w6966) -> ("error out"=w6987:errorcluster, "State Machine.lvclass"=w6988:refnum<class "State Machine.lvclass">, "Device out"=w6984:refnum<class "Channel.lvclass">)  [unwired: 7 in]
            n2878 = call "Next State.vi"("error in (no error)"=w6987, "New_State"=u32 35, "State Machine in"=w6988) -> ("error out"=w6982:errorcluster, "State Machine out"=w6985:refnum<class "State Machine.lvclass">)  [unwired: 7 in]
            n2879 = call-dynamic "Write State Machine.vi"("error in (no error)"=w6982, "State Machine.lvclass"=w6985, "Device in"=w6984) -> ("error out"=w6978:errorcluster, "Device out"=w6977:refnum<class "Channel.lvclass">)  [unwired: 7 in]
            n2880 = call-dynamic "Write Channel.vi"("error in (no error)"=w6978, "Channel.lvclass"=w6977, "Acquisition in"=w6983) -> ("error out"=w6979:errorcluster, "Acquisition out"=w6981:refnum<class "Acquisition.lvclass">)  [unwired: 7 in]
            n2881 = call-dynamic "Write AcquisitionA.vi"("error in (no error)"=w6979, "Acquisition.lvclass"=w6981, "S4ACS_GUI in"=w6980) -> ("error out"=w6974:errorcluster, "S4ACS_GUI out"=w6973:refnum<class "S4GUI.lvclass">)  [unwired: 7 in]
          }
        }
      }
      event "Set Temp 2": Value Change {
        n2882 = event-data() -> ("NewVal"=w6991:bool)  [unwired: 1 in]
        n2883 = case shown="True" w6991 {
          tunnel: w6995 -> [w6997 w7011]
          tunnel: w6994 -> [w6996 w7010]
          tunnel: [w6996 w7009] -> w6993
          tunnel: [w6997 w7008] -> w6992
          frame False {
          }
          frame True {
            n2884 = call "Read AcquisitionB.vi"("error in (no error)"=w7010, "S4ACS_GUI in"=w7011) -> ("error out"=w7024:errorcluster, "Acquisition.lvclass"=w7025:refnum<class "Acquisition.lvclass">, "S4ACS_GUI out"=w7015:refnum<class "S4GUI.lvclass">)  [unwired: 7 in]
            n2885 = call-dynamic "Read Channel.vi"("error in (no error)"=w7024, "Acquisition in"=w7025) -> ("error out"=w7006:errorcluster, "Channel.lvclass"=w7007:refnum<class "Channel.lvclass">, "Acquisition out"=w7018:refnum<class "Acquisition.lvclass">)  [unwired: 7 in]
            n2886 = call-dynamic "Read Interface.vi"("error in (no error)"=w7006, "Channel in"=w7007) -> ("error out"=w7004:errorcluster, "Interface.lvclass"=w7005:refnum<class "Interface.lvclass">, "Channel out"=w7002:refnum<class "Channel.lvclass">)  [unwired: 7 in]
            n2887 = call-dynamic "Write Temperature.vi"("error in (no error)"=w7004, "Temperature"="Target Temp 2", "Interface in"=w7005) -> ("error out"=w7000:errorcluster, "Interface out"=w7003:refnum<class "Interface.lvclass">)  [unwired: 7 in]
            n2888 = call-dynamic "Write Interface.vi"("error in (no error)"=w7000, "Interface.lvclass"=w7003, "Channel in"=w7002) -> ("error out"=w6999:errorcluster, "Channel out"=w7001:refnum<class "Channel.lvclass">)  [unwired: 7 in]
            n2889 = call-dynamic "Read State Machine.vi"("error in (no error)"=w6999, "Device in"=w7001) -> ("error out"=w7022:errorcluster, "State Machine.lvclass"=w7023:refnum<class "State Machine.lvclass">, "Device out"=w7019:refnum<class "Channel.lvclass">)  [unwired: 7 in]
            n2890 = call "Next State.vi"("error in (no error)"=w7022, "New_State"=u32 35, "State Machine in"=w7023) -> ("error out"=w7017:errorcluster, "State Machine out"=w7020:refnum<class "State Machine.lvclass">)  [unwired: 7 in]
            n2891 = call-dynamic "Write State Machine.vi"("error in (no error)"=w7017, "State Machine.lvclass"=w7020, "Device in"=w7019) -> ("error out"=w7013:errorcluster, "Device out"=w7012:refnum<class "Channel.lvclass">)  [unwired: 7 in]
            n2892 = call-dynamic "Write Channel.vi"("error in (no error)"=w7013, "Channel.lvclass"=w7012, "Acquisition in"=w7018) -> ("error out"=w7014:errorcluster, "Acquisition out"=w7016:refnum<class "Acquisition.lvclass">)  [unwired: 7 in]
            n2893 = call "Write AcquisitionB.vi"("error in (no error)"=w7014, "Acquisition.lvclass"=w7016, "S4ACS_GUI in"=w7015) -> ("error out"=w7009:errorcluster, "S4ACS_GUI out"=w7008:refnum<class "S4GUI.lvclass">)  [unwired: 7 in]
          }
        }
      }
      event "Set Temp 3": Value Change {
        n2894 = event-data() -> ("NewVal"=w7026:bool)  [unwired: 1 in]
        n2895 = case shown="True" w7026 {
          tunnel: w7030 -> [w7032 w7046]
          tunnel: w7029 -> [w7031 w7045]
          tunnel: [w7031 w7044] -> w7028
          tunnel: [w7032 w7043] -> w7027
          frame False {
          }
          frame True {
            n2896 = call-dynamic "Read AcquisitionC.vi"("error in (no error)"=w7045, "S4ACS_GUI in"=w7046) -> ("error out"=w7059:errorcluster, "Acquisition.lvclass"=w7060:refnum<class "Acquisition.lvclass">, "S4ACS_GUI out"=w7050:refnum<class "S4GUI.lvclass">)  [unwired: 7 in]
            n2897 = call-dynamic "Read Channel.vi"("error in (no error)"=w7059, "Acquisition in"=w7060) -> ("error out"=w7041:errorcluster, "Channel.lvclass"=w7042:refnum<class "Channel.lvclass">, "Acquisition out"=w7053:refnum<class "Acquisition.lvclass">)  [unwired: 7 in]
            n2898 = call-dynamic "Read Interface.vi"("error in (no error)"=w7041, "Channel in"=w7042) -> ("error out"=w7039:errorcluster, "Interface.lvclass"=w7040:refnum<class "Interface.lvclass">, "Channel out"=w7037:refnum<class "Channel.lvclass">)  [unwired: 7 in]
            n2899 = call-dynamic "Write Temperature.vi"("error in (no error)"=w7039, "Temperature"="Target Temp 3", "Interface in"=w7040) -> ("error out"=w7035:errorcluster, "Interface out"=w7038:refnum<class "Interface.lvclass">)  [unwired: 7 in]
            n2900 = call-dynamic "Write Interface.vi"("error in (no error)"=w7035, "Interface.lvclass"=w7038, "Channel in"=w7037) -> ("error out"=w7034:errorcluster, "Channel out"=w7036:refnum<class "Channel.lvclass">)  [unwired: 7 in]
            n2901 = call-dynamic "Read State Machine.vi"("error in (no error)"=w7034, "Device in"=w7036) -> ("error out"=w7057:errorcluster, "State Machine.lvclass"=w7058:refnum<class "State Machine.lvclass">, "Device out"=w7054:refnum<class "Channel.lvclass">)  [unwired: 7 in]
            n2902 = call "Next State.vi"("error in (no error)"=w7057, "New_State"=u32 35, "State Machine in"=w7058) -> ("error out"=w7052:errorcluster, "State Machine out"=w7055:refnum<class "State Machine.lvclass">)  [unwired: 7 in]
            n2903 = call-dynamic "Write State Machine.vi"("error in (no error)"=w7052, "State Machine.lvclass"=w7055, "Device in"=w7054) -> ("error out"=w7048:errorcluster, "Device out"=w7047:refnum<class "Channel.lvclass">)  [unwired: 7 in]
            n2904 = call-dynamic "Write Channel.vi"("error in (no error)"=w7048, "Channel.lvclass"=w7047, "Acquisition in"=w7053) -> ("error out"=w7049:errorcluster, "Acquisition out"=w7051:refnum<class "Acquisition.lvclass">)  [unwired: 7 in]
            n2905 = call-dynamic "Write AcquisitionC.vi"("error in (no error)"=w7049, "Acquisition.lvclass"=w7051, "S4ACS_GUI in"=w7050) -> ("error out"=w7044:errorcluster, "S4ACS_GUI out"=w7043:refnum<class "S4GUI.lvclass">)  [unwired: 7 in]
          }
        }
      }
      event "Set Temp 4": Value Change {
        n2906 = event-data() -> ("NewVal"=w7061:bool)  [unwired: 1 in]
        n2907 = case shown="True" w7061 {
          tunnel: w7065 -> [w7067 w7081]
          tunnel: w7064 -> [w7066 w7080]
          tunnel: [w7066 w7079] -> w7063
          tunnel: [w7067 w7078] -> w7062
          frame False {
          }
          frame True {
            n2908 = call-dynamic "Read AcquisitionD.vi"("error in (no error)"=w7080, "S4ACS_GUI in"=w7081) -> ("error out"=w7094:errorcluster, "Acquisition.lvclass"=w7095:refnum<class "Acquisition.lvclass">, "S4ACS_GUI out"=w7085:refnum<class "S4GUI.lvclass">)  [unwired: 7 in]
            n2909 = call-dynamic "Read Channel.vi"("error in (no error)"=w7094, "Acquisition in"=w7095) -> ("error out"=w7076:errorcluster, "Channel.lvclass"=w7077:refnum<class "Channel.lvclass">, "Acquisition out"=w7088:refnum<class "Acquisition.lvclass">)  [unwired: 7 in]
            n2910 = call-dynamic "Read Interface.vi"("error in (no error)"=w7076, "Channel in"=w7077) -> ("error out"=w7074:errorcluster, "Interface.lvclass"=w7075:refnum<class "Interface.lvclass">, "Channel out"=w7072:refnum<class "Channel.lvclass">)  [unwired: 7 in]
